vi "Request Detach.vi"(8 "error in (no error)":errorcluster, 10 "SensorView Enqueuer":refnum<class "Message Enqueuer.lvclass">, 11 "Sensor in":refnum<class "Sensor.lvclass">) -> (0 "error out":errorcluster, 3 "Sensor out":refnum<class "Sensor.lvclass">)   [LabVIEW 2012, in "Sensor Definition.lvlib" / "Sensor.lvclass"]
uses:
  Sensor.lvclass
  <vilib>/ActorFramework/Message Enqueuer/Message Enqueuer.lvclass
  Sensor.lvclass/Sensor.ctl
  HostType.ctl
  <vilib>/ActorFramework/Actor/Actor.lvclass/Actor.ctl
  <vilib>/ActorFramework/Message Enqueuer/Message Enqueuer.lvclass/Message Enqueuer.ctl
  Write Listening HostTypes.vi
  Read Listening HostTypes.vi
  Read Listening SensorViews.vi
  <vilib>/ActorFramework/Message Enqueuer/Enqueue.vi
  <vilib>/ActorFramework/Message Priority Queue/Priority Enqueue.vi
  DemoMain Messages/Detach MainPane Msg/Detach MainPane Msg.lvclass
  Sensor Definition.lvlib
  <vilib>/ActorFramework/Actor/Actor.lvclass
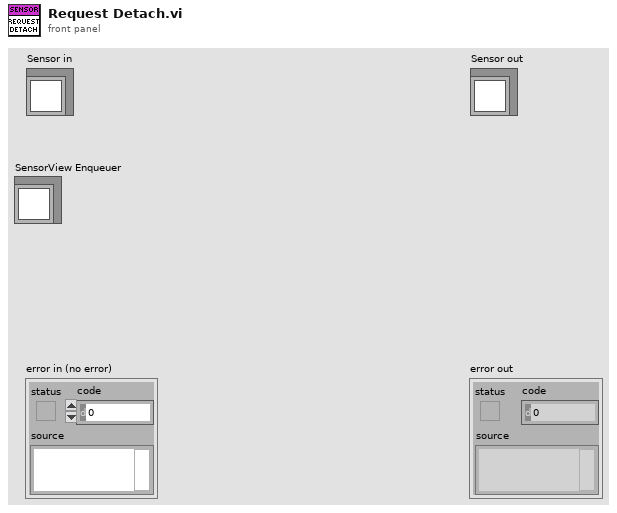
[diagram p1: front panel]
types:
  T1 = typedef "Sensor Definition.lvlib/HostType.ctl" = enum16{"Standalone", "Grid", "MainPane"}
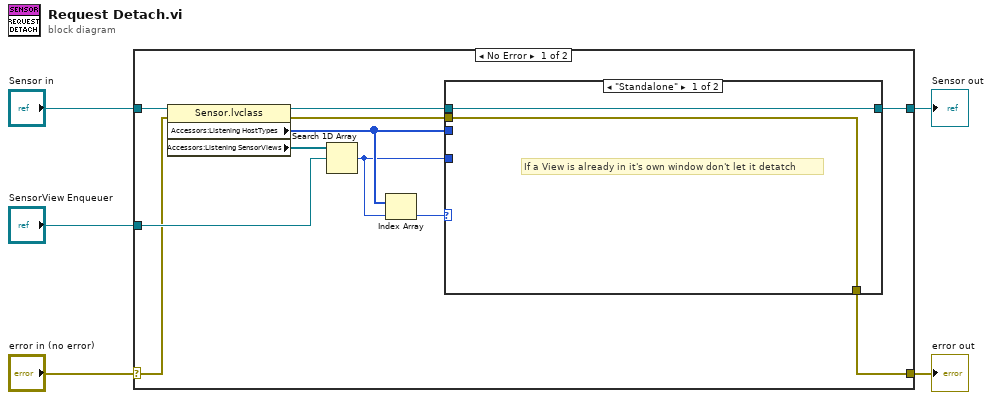
[diagram p0: block diagram]
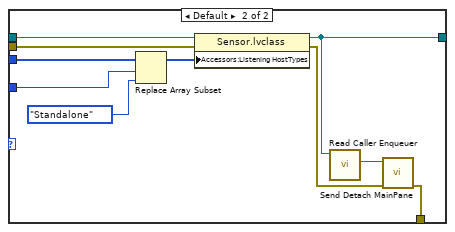
[diagram p2: hidden frame]
diagram:
  n1 = case shown="No Error" "error in (no error)" {
    selector: "error in (no error)" -> [w11 w30]
    tunnel: [w9 w30] -> w4
    tunnel: [w12 w29] -> w2
    tunnel: "Sensor in" -> [w16 w29]
    tunnel: "SensorView Enqueuer" -> [w13 _]
    frame No Error {
      n2 = property class="Sensor.lvclass"(reference=w16, error in=w11) -> (reference out=w15:refnum<class "Sensor.lvclass">, error out=w10:errorcluster, "Accessors:Listening HostTypes"=w8:T1[], "Accessors:Listening SensorViews"=w14:refnum<class "Message Enqueuer.lvclass">[])
      n3 = Search 1D Array(1D array=w14, element=w13) -> (index of element=w7:i32)  [unwired: 1 in]
      n4 = Index Array(array=w8, index=w7) -> (element=w6:T1)
      n5 = case shown="\"Standalone\"" w6 {
        tunnel: w15 -> [w18 w28]
        tunnel: w8 -> [_ w27]
        tunnel: w7 -> [_ w26]
        tunnel: [w18 w23] -> w12
        tunnel: w10 -> [w17 w21]
        tunnel: [w17 w19] -> w9
        frame "Standalone" {
          # "If a View is already in it's own window don't let it detatch"
        }
        frame Default {
          n6 = Replace Array Subset(array=w27, new element=HostType."Standalone" ("new element/subarray"), index=w26) -> (w25:T1[])
          n7 = property class="Sensor.lvclass"(reference=w28, error in=w21, "Accessors:Listening HostTypes"=w25) -> (reference out=w23:refnum<class "Sensor.lvclass">, error out=w20:errorcluster)
          n8 = call <vilib>:"Read Caller Enqueuer.vi"("Actor"=w23) -> ("Caller Enqueuer"=w22:refnum<class "Message Enqueuer.lvclass">)  [unwired: 10 in]
          n9 = call "Send Detach MainPane.vi"("error in (no error)"=w20, "Message Enqueuer"=w22) -> ("error out"=w19:errorcluster)  [unwired: 8 in, 1 out]
        }
      }
    }
    frame Error {
    }
  }
  "error out" <- w4
  "Sensor out" <- w2
